vi "sftp_statvfs.vi"() -> ()   [LabVIEW 2013]
doc: "Illustrates how to read file system statistics from a remote SFTP server."
uses:
  libssh2/libssh2_sftp_statvfs.ctl
  libssh2/libssh2_init_default.vi
  libssh2/libssh2_session_handshake_tcp.vi
  libssh2/libssh2.lvlib
panel:
  in  "Method":enum16{"statvfs", "fstatvfs"}(ring)
  in  "path":string="/"
  out "available space in GiB":dbl
  out "free space in GiB":dbl
  out "size in GiB":dbl
  out "statvfs":T1
  out "error out":errorcluster
  in  "password":string
  in  "username":string
  in  "hostname":string
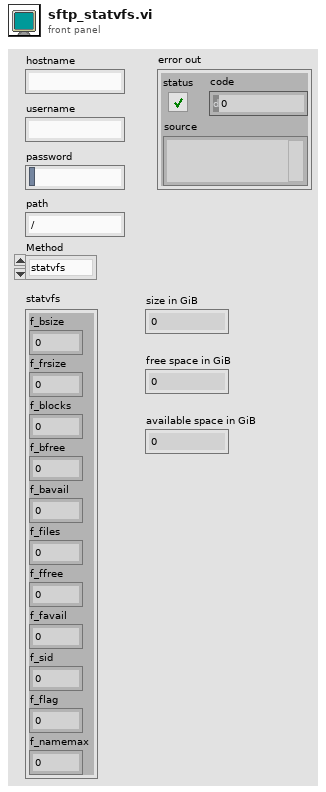
[diagram p1: front panel]
types:
  T1 = typedef "libssh2.lvlib/libssh2_sftp_statvfs.ctl" = cluster{"f_bsize":u64, "f_frsize":u64, "f_blocks":u64, "f_bfree":u64, "f_bavail":u64, "f_files":u64, "f_ffree":u64, "f_favail":u64, "f_sid":u64, "f_flag":u64, "f_namemax":u64}
  T2 = typedef "libssh2.lvlib/Session Refnum.ctl" = refnum<k1>
  T3 = typedef "libssh2.lvlib/SFTP Refnum.ctl" = refnum<k1>
  T4 = typedef "libssh2.lvlib/SFTP Handle Refnum.ctl" = refnum<k1>
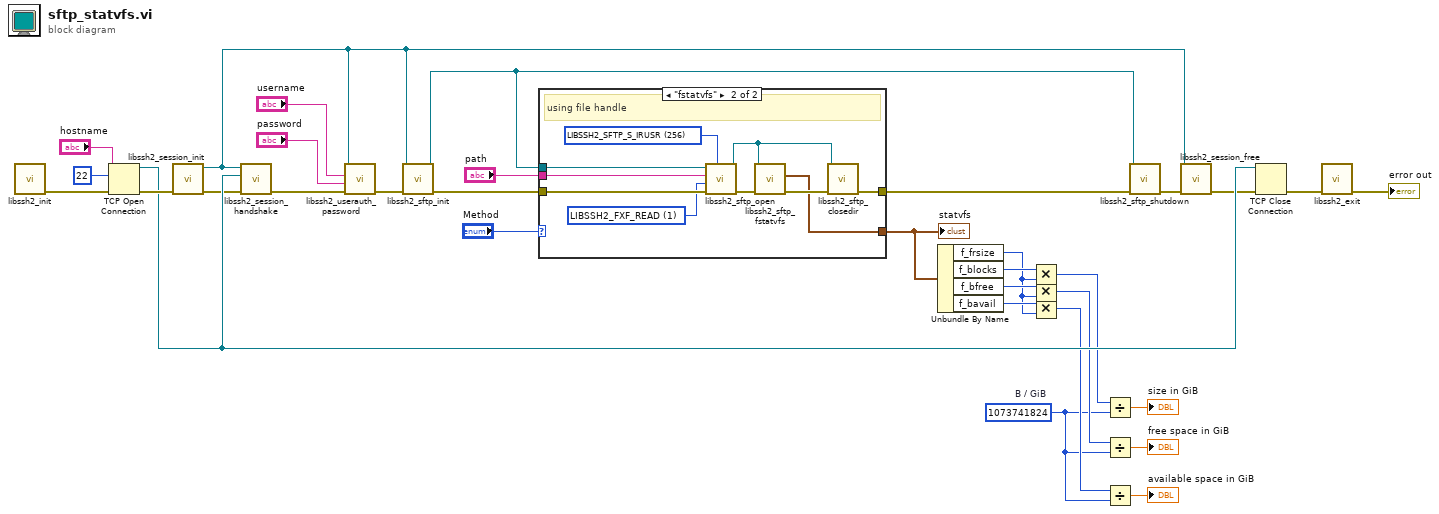
[diagram p0: block diagram]
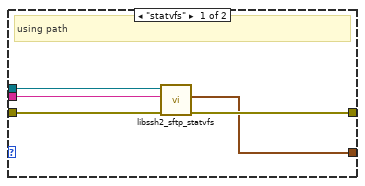
[diagram p2: hidden frame]
diagram:
  w2 = u64 1073741824  # B / GiB
  n1 = call-poly "libssh2_init.vi"() -> ("error out"=w31:errorcluster)  [unwired: 11 in]
  n2 = TCP Open Connection(address="hostname", remote port or service name=u16 22, error in (no error)=w31) -> (connection ID=w29:refnum<k5>, error out=w30:errorcluster)  [unwired: 2 in]
  n3 = call "libssh2_session_init.vi"("error in (no error)"=w30) -> ("error out"=w28:errorcluster, "session"=w21:T2)  [unwired: 9 in]
  n4 = call-poly "libssh2_session_handshake.vi"("error in (no error)"=w28, "tcp connection"=w29, "session"=w21) -> ("error out"=w32:errorcluster)  [unwired: 8 in]
  n5 = call "libssh2_userauth_password.vi"("error in (no error)"=w32, "password"="password", "username"="username", "session"=w21) -> ("error out"=w25:errorcluster)  [unwired: 7 in]
  n6 = call "libssh2_sftp_init.vi"("error in (no error)"=w25, "session"=w21) -> ("error out"=w17:errorcluster, "sftp"=w15:T3)  [unwired: 8 in]
  n7 = case shown="\"fstatvfs\"" "Method" {
    tunnel: w17 -> [w37 w47]
    tunnel: [w36 w43] -> w16
    tunnel: w15 -> [w35 w45]
    tunnel: "path" -> [w34 w44]
    tunnel: [w33 w40] -> w13
    frame "statvfs" {
      # "using path"
      n8 = call "libssh2_sftp_statvfs.vi"("error in (no error)"=w37, "path"=w34, "sftp"=w35) -> ("error out"=w36:errorcluster, "statvfs"=w33:T1)  [unwired: 7 in]
    }
    frame "fstatvfs" {
      w38 = u32 1 items=["LIBSSH2_FXF_READ"=1, "LIBSSH2_FXF_WRITE"=2, "LIBSSH2_FXF_APPEND"=4, "LIBSSH2_FXF_CREAT"=8, "LIBSSH2_FXF_TRUNC"=16, "LIBSSH2_FXF_EXCL"=32] ("flags")
      w39 = 256 items=["LIBSSH2_SFTP_S_IRWXU"=448, "LIBSSH2_SFTP_S_IRUSR"=256, "LIBSSH2_SFTP_S_IWUSR"=128, "LIBSSH2_SFTP_S_IXUSR"=64, "LIBSSH2_SFTP_S_IRWXG"=56, "LIBSSH2_SFTP_S_IRGRP"=32, "LIBSSH2_SFTP_S_IWGRP"=16, "LIBSSH2_SFTP_S_IXGRP"=8, "LIBSSH2_SFTP_S_IRWXO"=7, "LIBSSH2_SFTP_S_IROTH"=4, "LIBSSH2_SFTP_S_IWOTH"=2, "LIBSSH2_SFTP_S_IXOTH"=1] ("mode")
      # "using file handle"
      n9 = call "libssh2_sftp_open.vi"("mode"=w39, "error in (no error)"=w47, "flags"=w38, "path"=w44, "sftp"=w45) -> ("error out"=w46:errorcluster, "sftp handle"=w41:T4)  [unwired: 5 in]
      n10 = call "libssh2_sftp_fstatvfs.vi"("error in (no error)"=w46, "sftp handle"=w41) -> ("error out"=w42:errorcluster, "statvfs"=w40:T1)  [unwired: 8 in]
      n11 = call "libssh2_sftp_closedir.vi"("error in (no error)"=w42, "sftp handle"=w41) -> ("error out"=w43:errorcluster)  [unwired: 9 in]
    }
  }
  "statvfs" <- w13
  n12 = Unbundle By Name(w13) -> ("f_frsize"=w4:u64, "f_blocks"=w12:u64, "f_bfree"=w9:u64, "f_bavail"=w5:u64)
  n13 = Multiply(x=w12, y=w4) -> (x*y=w11:u64)
  n14 = Multiply(x=w9, y=w4) -> (x*y=w7:u64)
  n15 = Multiply(x=w5, y=w4) -> (x*y=w3:u64)
  n16 = Divide(x=w11, y=w2) -> (x/y=→"size in GiB":dbl)
  n17 = Divide(x=w7, y=w2) -> (x/y=→"free space in GiB":dbl)
  n18 = Divide(x=w3, y=w2) -> (x/y=→"available space in GiB":dbl)
  n19 = call "libssh2_sftp_shutdown.vi"("error in (no error)"=w16, "sftp"=w15) -> ("error out"=w18:errorcluster)  [unwired: 9 in]
  n20 = call "libssh2_session_free.vi"("error in (no error)"=w18, "session"=w21) -> ("error out"=w20:errorcluster)  [unwired: 9 in]
  n21 = TCP Close Connection(connection ID=w29, error in (no error)=w20) -> (error out=w19:errorcluster)  [unwired: 1 in, 1 out]
  n22 = call "libssh2_exit.vi"("error in (no error)"=w19) -> ("error out"=→"error out":errorcluster)  [unwired: 10 in]
